vi "DigitalDisplayVisible.vi"(6 "error in":errorcluster, 9 "Knob in":refnum<class "Knob.lvclass">) -> (0 "error out":errorcluster, 3 "Knob out":refnum<class "Knob.lvclass">, 4 "digital display":bool)   [LabVIEW 2014, in "Knob.lvclass"]
uses:
  Knob.lvclass
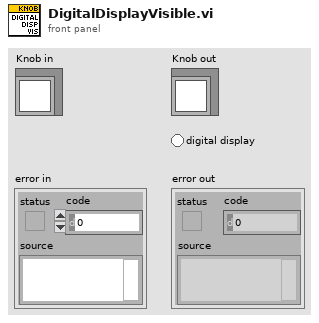
[diagram p1: front panel]
types:
  T1 = typedef "LVRectTypeDef.ctl" = cluster{"Left":i16, "Top":i16, "Right":i16, "Bottom":i16}
  T2 = cluster{"left":i16, "top":i16, "right":i16, "bottom":i16}
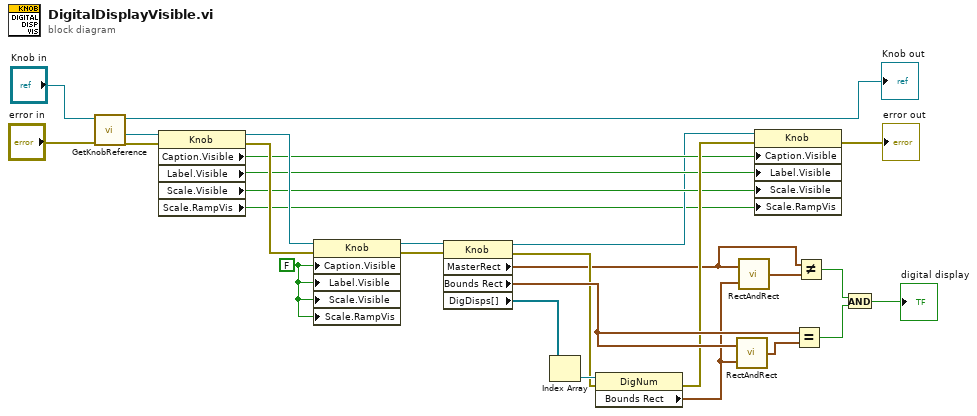
[diagram p0: block diagram]
diagram:
  w2 = FALSE ("Caption.Visible")
  n1 = call "GetKnobReference.vi"("error in"="error in", "Knob in"="Knob in") -> ("error out"=w8:errorcluster, "knob reference"=w9:refnum<vi>, "Knob out"=→"Knob out":refnum<class "Knob.lvclass">)  [unwired: 7 in]
  n2 = property class="Knob"(reference=w9, error in=w8) -> (reference out=w22:refnum<vi>, error out=w21:errorcluster, "Caption.Visible"=w16:bool, "Label.Visible"=w15:bool, "Scale.Visible"=w14:bool, "Scale.RampVis"=w1:bool)
  n3 = property class="Knob"(reference=w22, error in=w21, "Caption.Visible"=w2, "Label.Visible"=w2, "Scale.Visible"=w2, "Scale.RampVis"=w2) -> (reference out=w20:refnum<vi>, error out=w19:errorcluster)
  n4 = property class="Knob"(reference=w20, error in=w19) -> (reference out=w13:refnum<vi>, error out=w18:errorcluster, "MasterRect"=w12:T1, "Bounds Rect"=w25:T1, "DigDisps[]"=w28:refnum<vi>[])
  n5 = Index Array(array=w28) -> (element=w27:refnum<vi>)  [unwired: 1 in]
  n6 = property class="DigNum"(reference=w27, error in=w18) -> (error out=w17:errorcluster, "Bounds Rect"=w24:T1)  [unwired: 1 out]
  n7 = call <vilib>:"RectAndRect.vi"("rect b"=w24, "rect a"=w25) -> ("union rect"=w26:T2)
  n8 = call <vilib>:"RectAndRect.vi"("rect b"=w24, "rect a"=w12) -> ("union rect"=w23:T2)
  n9 = property class="Knob"(reference=w13, error in=w17, "Caption.Visible"=w16, "Label.Visible"=w15, "Scale.Visible"=w14, "Scale.RampVis"=w1) -> (error out=→"error out":errorcluster)  [unwired: 1 out]
  n10 = Equal?(x=w25, y=w26) -> (x = y?=w10:bool)
  n11 = Not Equal?(x=w12, y=w23) -> (x != y?=w11:bool)
  n12 = And(x=w11, y=w10) -> (x .and. y?=→"digital display":bool)
